vi "LZ-DataInitial.vi"() -> (3 "数据 初始化":string[][](table))   [LabVIEW 2015]
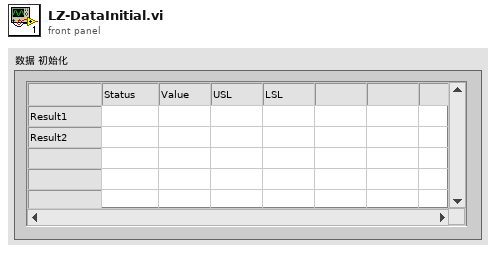
[diagram p1: front panel]
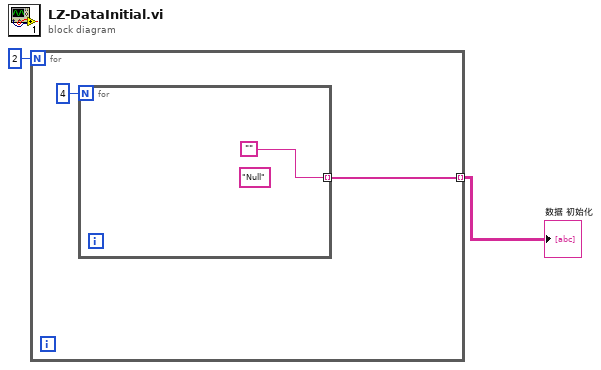
[diagram p0: block diagram]
diagram:
  n1 = for {
    N: 2 -> [_]
    tunnel: [w4] -> w2 mode=indexing
    n2 = for {
      N: 4 -> [_]
      tunnel: [""] -> w4 mode=indexing
      (unwired) "Null"
    }
  }
  "数据 初始化" <- w2
